vi "__uintSetBaseUint.vi"(8 "Error in (no error)":errorcluster, 9 "Base (decimal)":T1=10 items=["Binary"=2, "Octal"=8, "Decimal"=10, "Hexadecimal"=16, "Hexatrigesimal"=36, "ASCII"=64], 10 "Uint in":u8[](array[numeric])=[0], 11 "Uint in":refnum<class "UintClass.lvclass">) -> (0 "error out":errorcluster, 3 "Uint out":refnum<class "UintClass.lvclass">)   [LabVIEW 2011]
uses:
  enumBase.ctl
  UintClass.lvclass
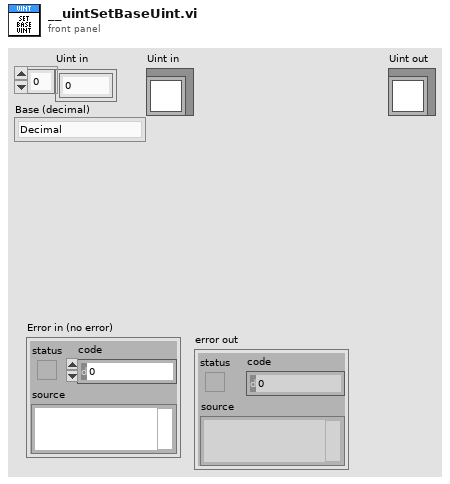
[diagram p1: front panel]
types:
  T1 = typedef "UintClass.lvclass/enumBase.ctl" = u16
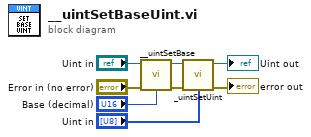
[diagram p0: block diagram]
diagram:
  n1 = call "__uintSetBase.vi"("Error in (no error)"="Error in (no error)", "Base (decimal)"="Base (decimal)", "Uint in"="Uint in") -> ("Error out"=w1:errorcluster, "Uint out"=w2:refnum<class "UintClass.lvclass">)  [unwired: 7 in]
  n2 = call "_uintSetUint.vi"("Error in (no error)"=w1, 10:"Uint in"="Uint in", 11:"Uint in"=w2) -> ("Error out"=→"error out":errorcluster, "Uint out"=→"Uint out":refnum<class "UintClass.lvclass">)  [unwired: 7 in]
